vi "Find Line through Grid.vi"(9 "Point 2":cluster{"Obj X":dbl, "Obj Y":dbl}, 10 "Point 1":cluster{"Robot X (m)":dbl, "Robot Y (m)":dbl}, 11 "Grid Settings":T1={"X cells"=40, "Y cells"=40, "X size (m)"=0.1, "Y size (m)"=0.1}) -> (3 "Array":cluster{"x":i32, "y":i32}[](array[cluster]))   [LabVIEW 2012]
panel:
  out "Line Equation":cluster{"m":dbl, "c":dbl}
  # "Outputs an array of cells between object and\nrobot."
  # "Debugging. Equation found for line"
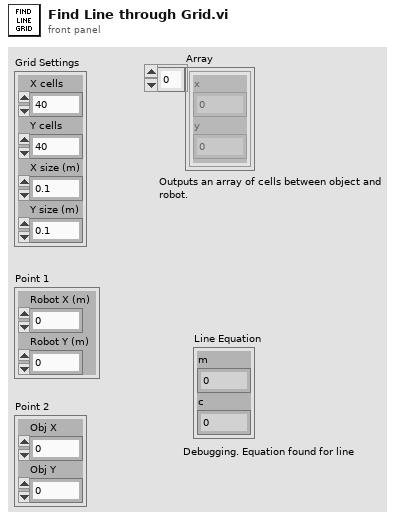
[diagram p1: front panel]
types:
  T1 = cluster{"X cells":i32, "Y cells":i32, "X size (m)":dbl, "Y size (m)":dbl}
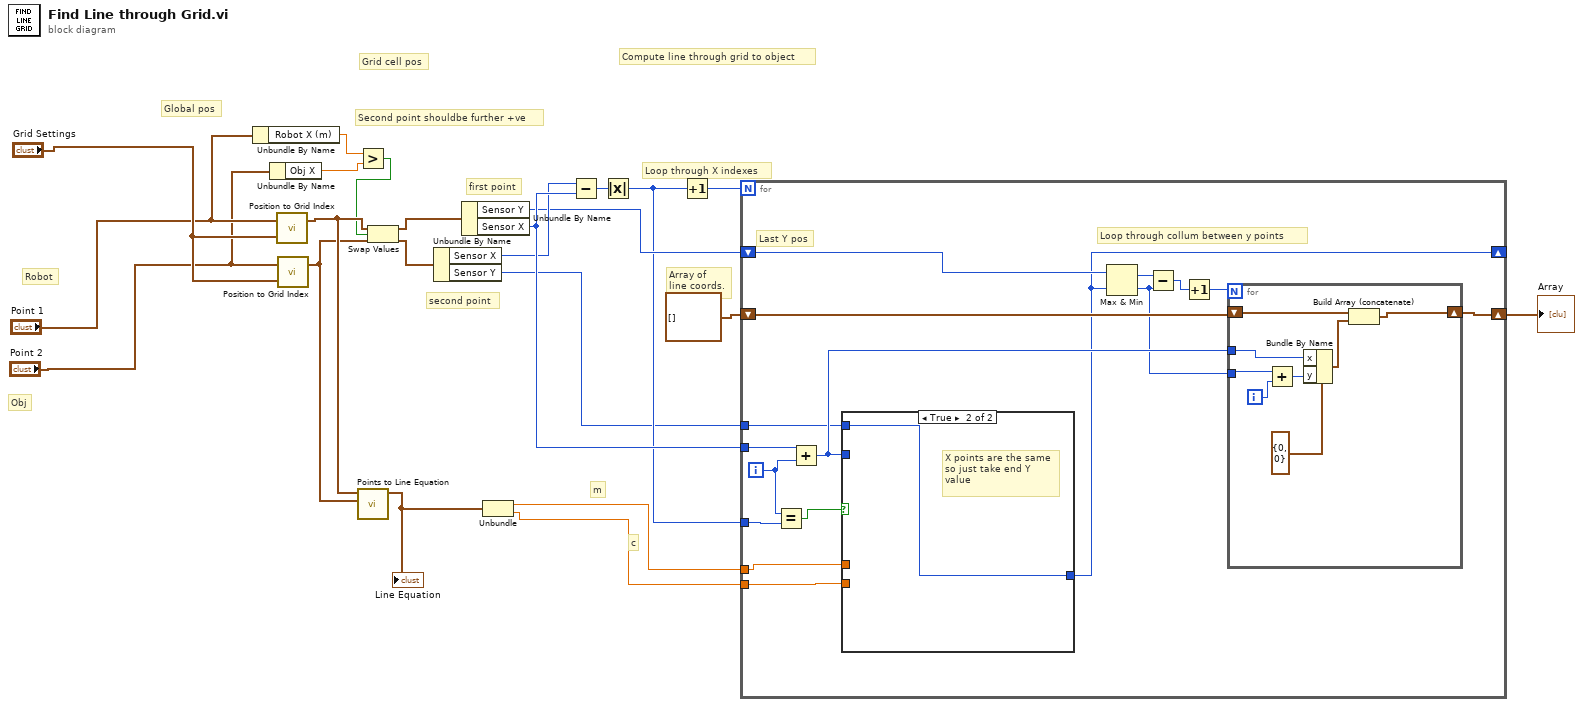
[diagram p0: block diagram]
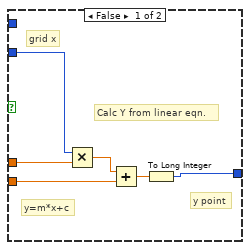
[diagram p2: hidden frame]
diagram:
  # "Second point shouldbe further +ve"
  # "second point"
  # "first point"
  # "Array of\nline coords."
  # "Global pos"
  # "Obj"
  # "Robot"
  # "c"
  # "m"
  # "Loop through X indexes"
  # "Compute line through grid to object"
  # "Grid cell pos"
  n1 = Unbundle By Name("Point 1") -> ("Robot X (m)"=w10:dbl)
  n2 = Unbundle By Name("Point 2") -> ("Obj X"=w9:dbl)
  n3 = call "Position to Grid Index.vi"("Grid Settings"="Grid Settings", "Global Position"="Point 1") -> ("Grid Index"=w6:cluster{"Sensor X":i32, "Sensor Y":i32})  [unwired: 1 out]
  n4 = call "Position to Grid Index.vi"("Grid Settings"="Grid Settings", "Global Position"="Point 2") -> ("Grid Index"=w5:cluster{"Sensor X":i32, "Sensor Y":i32})  [unwired: 1 out]
  n5 = Greater?(x=w10, y=w9) -> (0:w4:bool)
  n6 = call "Points to Line Equation.vi"("Point 2"=w5, "Point 1"=w6) -> ("Line Equation"=w14:cluster{"m":dbl, "c":dbl})  [unwired: 9 in]
  "Line Equation" <- w14
  n7 = Swap Values(12:w6, 13:w4, 14:w5) -> (1:w8:cluster{"Sensor X":i32, "Sensor Y":i32}, 3:w7:cluster{"Sensor X":i32, "Sensor Y":i32})
  n8 = Unbundle By Name(w7) -> ("Sensor X"=w18:i32, "Sensor Y"=w1:i32)
  n9 = Unbundle By Name(w8) -> ("Sensor Y"=w3:i32, "Sensor X"=w19:i32)
  n10 = Unbundle(w14) -> ("m"=w16:dbl, "c"=w15:dbl)
  n11 = Subtract(x=w18, y=w19) -> (x-y=w13:i32)
  n12 = Absolute Value(x=w13) -> (abs(x)=w2:i32)
  n13 = Increment(x=w2) -> (x+1=w22:i32)
  n14 = for {
    N: w22 -> [_]
    tunnel: w16 -> [w38]
    tunnel: w15 -> [w37]
    shift-right: [w25] -> _
    shift-left: w3 -> [w26]
    tunnel: w19 -> [w36]
    shift-right: [w34] -> w20
    shift-left: cluster{"x":i32, "y":i32}[] [] -> [w35]
    tunnel: w1 -> [w30]
    tunnel: w2 -> [w27]
    i -> [w29]
    # "Last Y pos"
    # "Loop through collum between y points"
    n15 = Equal?(x=w29, y=w27) -> (x = y?=w28:bool)
    n16 = Add(x=w36, y=w29) -> (x+y=w33:i32)
    n17 = case shown="True" w28 {
      tunnel: w38 -> [w44 _]
      tunnel: w37 -> [w42 _]
      tunnel: w33 -> [w40 _]
      tunnel: [w39 w45] -> w25
      tunnel: w30 -> [_ w45]
      frame False {
        # "Calc Y from linear eqn."
        # "grid x"
        # "y point"
        # "y=m*x+c"
        n18 = Multiply(x=w40, y=w44) -> (x*y=w43:dbl)
        n19 = Add(x=w43, y=w42) -> (x+y=w41:dbl)
        n20 = To Long Integer(number=w41) -> (32bit integer=w39:i32)
      }
      frame True {
        # "X points are the same\nso just take end Y\nvalue"
      }
    }
    n21 = Max & Min(x=w26, y=w25) -> (max(x,y)=w24:i32, min(x,y)=w23:i32)
    n22 = Subtract(x=w24, y=w23) -> (x-y=w32:i32)
    n23 = Increment(x=w32) -> (x+1=w31:i32)
    n24 = for {
      N: w31 -> [_]
      tunnel: w23 -> [w47]
      shift-right: [w52] -> w34
      shift-left: w35 -> [w53]
      tunnel: w33 -> [w51]
      i -> [w46]
      n25 = Add(x=w47, y=w46) -> (x+y=w48:i32)
      n26 = Bundle By Name(cluster=cluster{"x":i32, "y":i32} {"x"=0, "y"=0} ("grid index"), "x"=w51, "y"=w48) -> (w50:cluster{"x":i32, "y":i32})
      n27 = Build Array (concatenate)(w53, w50) -> (w52:cluster{"x":i32, "y":i32}[])
    }
  }
  "Array" <- w20
